vi "Distance.vi"(11 "Velocity":dbl[][](array[numeric])) -> (3 "Distance":dbl[][](array[numeric]))   [LabVIEW 2016]
uses:
  <vilib>/Analysis/NI_AALPro.lvlib
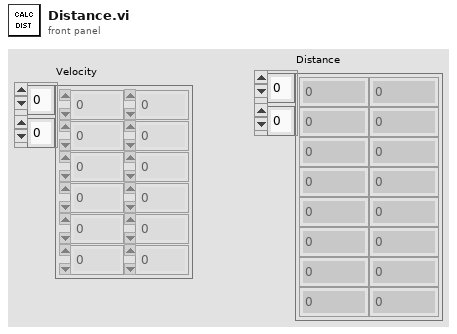
[diagram p1: front panel]
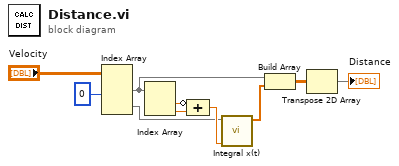
[diagram p0: block diagram]
diagram:
  n1 = Index Array(array="Velocity", index (col) #1=0 ("disabled index (col)")) -> (element #1=w6:dbl[], element #2=w3:dbl[])  [unwired: 3 in]
  n2 = Index Array(array=w6) -> (element #1=w9:dbl, element #2=w8:dbl)  [unwired: 2 in]
  n3 = Compound Arithmetic op=ADD(invert w9, w8) -> (w7:dbl)
  n4 = call <vilib>:"Integral x(t).vi"("dt"=w7, "X"=w3) -> ("Integral X"=w2:dbl[])  [unwired: 8 in, 1 out]
  n5 = Build Array(w6, w2) -> (w5:dbl[][])
  n6 = Transpose 2D Array(2D array=w5) -> (transposed array=→"Distance":dbl[][])
